vi "mupLib EvalMulti example.vi"() -> ()   [LabVIEW 2015]
uses:
  mupLib/mupLibPath.vi
  mupLib/mupCheckError.vi
  <vilib>/Utility/error.llb/Error Cluster From Error Code.vi
  mupLib/mupLib.lvlib
panel:
  out "error out":errorcluster
  out "Results":dbl[](array[numeric])
  in  "c":dbl=2.0
  in  "Expression":string="a*x^2+b*x+c,\n52,\na*sin(b*x+c)"
  in  "x":dbl=1.0
  in  "b":dbl=0.25
  in  "a":dbl=1.0
  # "Constants"
  # "Variables"
  # "This example demonstrates multi-expression evaluation using mupLib.\n\n- Enter multiple expressions using constants a, b, c and variable x\n- Enter the values of constants a, b, c\n- Enter the value of variable x\n- Hit run to evaluate all expressions."
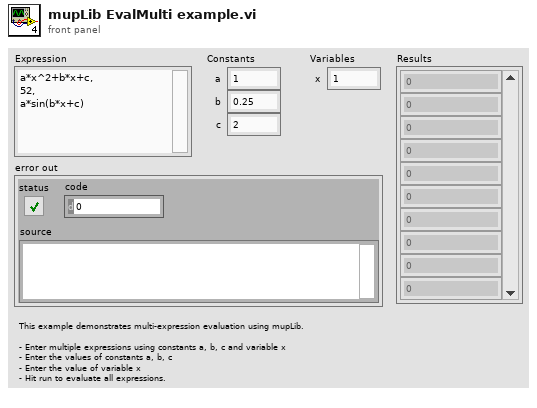
[diagram p1: front panel]
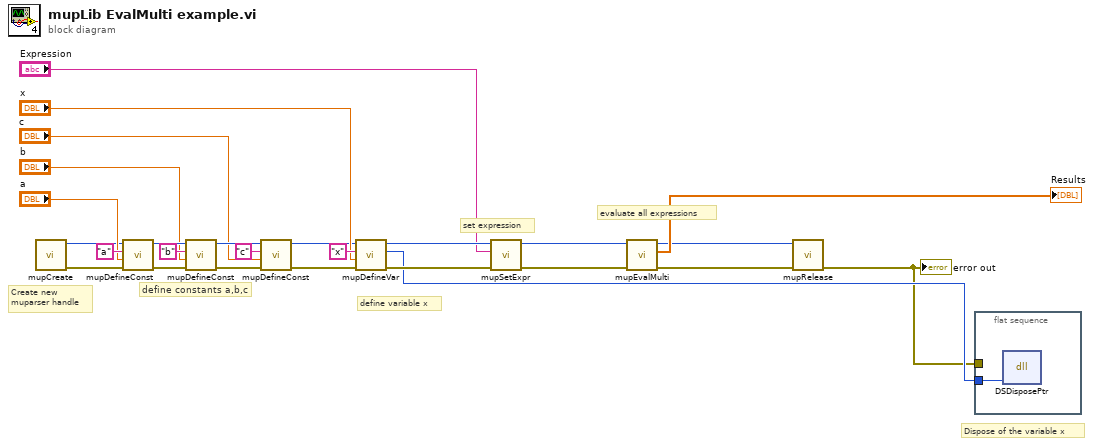
[diagram p0: block diagram]
diagram:
  # "evaluate all expressions"
  # "Dispose of the variable x"
  # "set expression"
  # "define variable x"
  # "define constants a,b,c"
  # "Create new\nmuparser handle"
  n1 = call "mupCreate.vi"() -> ("error out"=w26:errorcluster, "hParser out"=w8:u64)  [unwired: 10 in]
  n2 = call "mupDefineConst.vi"("error in (no error)"=w26, "Value"="a", "constName"="a", "hParser in"=w8) -> ("error out"=w21:errorcluster, "hParser out"=w22:u64)  [unwired: 6 in]
  n3 = call "mupDefineConst.vi"("error in (no error)"=w21, "Value"="b", "constName"="b", "hParser in"=w22) -> ("error out"=w12:errorcluster, "hParser out"=w13:u64)  [unwired: 6 in]
  n4 = call "mupDefineConst.vi"("error in (no error)"=w12, "Value"="c", "constName"="c", "hParser in"=w13) -> ("error out"=w10:errorcluster, "hParser out"=w9:u64)  [unwired: 6 in]
  n5 = call "mupDefineVar.vi"("error in (no error)"=w10, "initValue"="x", "varName"="x", "hParser in"=w9) -> ("error out"=w15:errorcluster, "varAddr"=w7:u64, "hParser out"=w17:u64)  [unwired: 5 in]
  n6 = call "mupSetExpr.vi"("error in (no error)"=w15, "szExpr"="Expression", "muPar in"=w17) -> ("error out"=w5:errorcluster, "muPar out"=w6:u64)  [unwired: 7 in]
  n7 = call "mupEvalMulti.vi"("error in (no error)"=w5, "hParser in"=w6) -> ("error out"=w2:errorcluster, "results"=→"Results":dbl[], "hParser out"=w3:u64)  [unwired: 6 in, 1 out]
  n8 = call "mupRelease.vi"("error in (no error)"=w2, "hParser in"=w3) -> ("error out"=w1:errorcluster)  [unwired: 9 in]
  "error out" <- w1
  n9 = flat-sequence {
    tunnel: w7 -> [w27]
    tunnel: w1 -> [_]
    frame #0 {
      n10 = dll-call lib="LabVIEW" fn="DSDisposePtr"("ptr"=w27) -> ()  [unwired: 5 in, 2 out]
    }
  }
